vi "Add Topic.vi"(8 "error in (no error)":errorcluster, 9 "Topic Enqueuer":refnum<class "Message Enqueuer.lvclass">, 10 "Topic Object":refnum<class "Topic.lvclass">, 11 "TopicLookupTable":refnum<data-value>) -> (0 "error out":errorcluster, 2 "Topic Replaced?":bool, 3 "TopicLookupTable":refnum<data-value>)   [LabVIEW 2015, in "Mediator.lvlib" / "TopicLookupTable.lvclass"]
doc: "<License>\nCopyright © 2017 Composed Systems, LLC | All rights reserved\nwww.composed.io\n\nAuthor: Ethan Stern <ethan.stern@composed.io>\n\nThis software is provided \"AS IS\" WITHOUT WARRANTIES, either express or implied, AND IS FOR EDUCATIONAL PURPOSES ONLY.\n</License>"
uses:
  TopicLookupTable.lvclass
  Topic/Topic.lvclass
  <vilib>/ActorFramework/Message Enqueuer/Message Enqueuer.lvclass
  Topic/Topic.lvclass/Topic.ctl
  TopicLookupTable.lvclass/TopicLookupTable.ctl
  <vilib>/ErrorRing/Error Ring.xnode
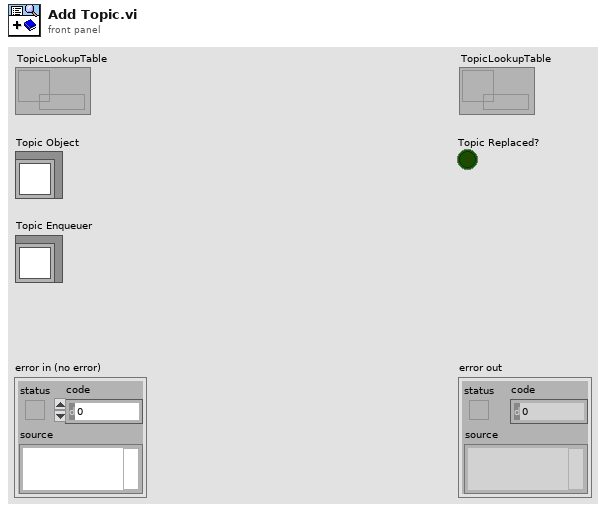
[diagram p1: front panel]
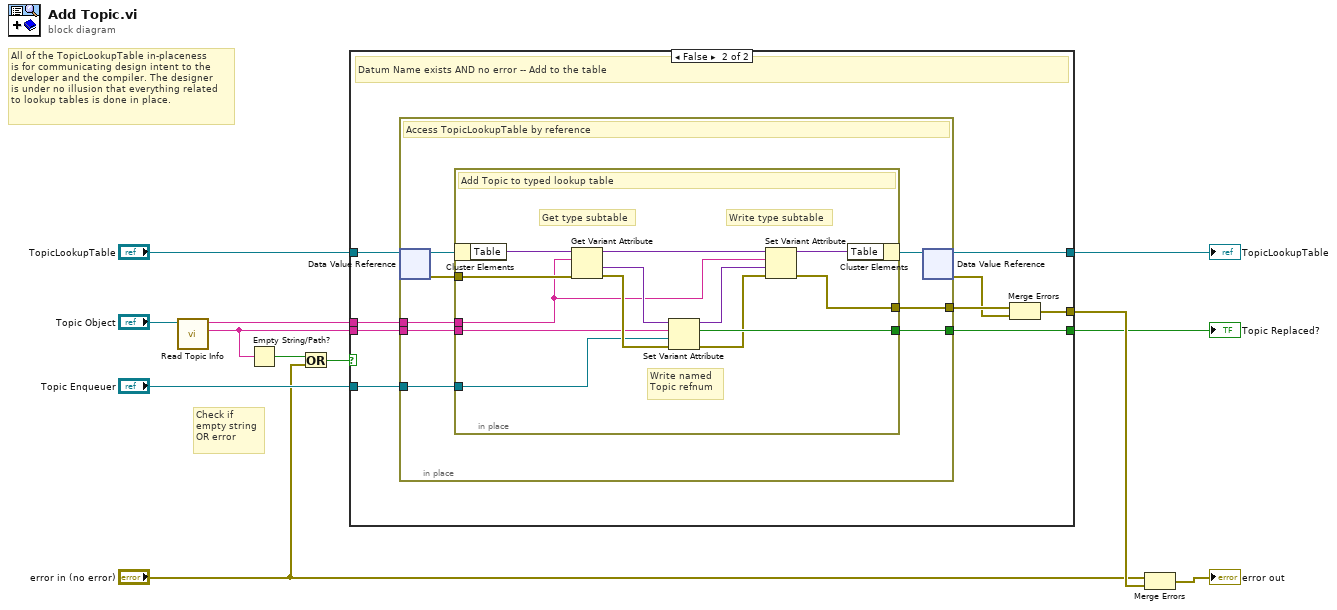
[diagram p0: block diagram]
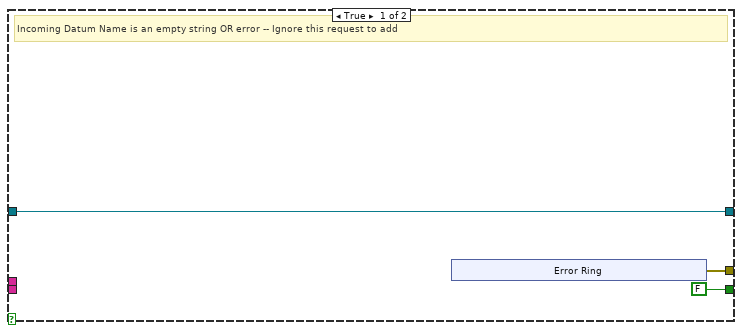
[diagram p2: hidden frame]
diagram:
  # "Check if\nempty string\nOR error"
  # "All of the TopicLookupTable in-placeness\nis for communicating design intent to the\ndeveloper and the compiler. The designer\nis under no illusion that everything related\nto lookup tables is done in place."
  n1 = call "Read Topic Info.vi"("Topic in"="Topic Object") -> ("Name"=w2:string, "Type"=w6:string)  [unwired: 7 in, 2 out]
  n2 = Empty String/Path?(string/path=w2) -> (empty?=w3:bool)
  n3 = Or(x=w3, y="error in (no error)") -> (x .or. y?=w1:bool)
  n4 = case shown="False" w1 {
    tunnel: "TopicLookupTable" -> [w13 w21]
    tunnel: [w14 w20] -> w10
    tunnel: [FALSE ("replaced") w24] -> w9
    tunnel: "Topic Enqueuer" -> [_ w23]
    tunnel: w6 -> [_ w22]
    tunnel: [w13 w18] -> w5
    tunnel: w2 -> [_ w17]
    frame True {
      # "Incoming Datum Name is an empty string OR error -- Ignore this request to add"
      n5 = xnode "Error Ring"() -> ("error out"=w14:errorcluster)
    }
    frame False {
      # "Datum Name exists AND no error -- Add to the table"
      n6 = in-place {
        in-place-border: [w33] -> w25
        in-place-border: [w32] -> w24
        in-place-border: w23 -> [w31]
        in-place-border: w22 -> [w30]
        in-place-border: w17 -> [w29]
        # "Access TopicLookupTable by reference"
        n7 = in-place-dvr #1(w21) -> (w28:refnum<class "TopicLookupTable.lvclass">, w26:errorcluster)
        n8 = in-place {
          in-place-border: [w44] -> w33
          in-place-border: [w39] -> w32
          in-place-border: w31 -> [w37]
          in-place-border: w30 -> [w34]
          in-place-border: w29 -> [w36]
          in-place-border: w26 -> [w35]
          # "Write named\nTopic refnum"
          # "Write type subtable"
          # "Get type subtable"
          # "Add Topic to typed lookup table"
          n9 = in-place-cluster #2(w28) -> ("Table"=w43:variant)
          n10 = Get Variant Attribute(Variant=w43, name=w34, error in=w35) -> (duplicate Variant=w42:variant, value=w40:variant, error out=w46:errorcluster)  [unwired: 1 in, 1 out]
          n11 = Set Variant Attribute(Variant=w40, name=w36, value=w37, error in=w46) -> (Variant out=w41:variant, replaced=w39:bool, error out=w38:errorcluster)
          n12 = Set Variant Attribute(Variant=w42, name=w34, value=w41, error in=w38) -> (Variant out=w45:variant, error out=w44:errorcluster)  [unwired: 1 out]
          n13 = in-place-cluster #2("Table"=w45) -> (w27:refnum<class "TopicLookupTable.lvclass">)
        }
        n14 = in-place-dvr #1(w27) -> (w18:refnum<data-value>, w19:errorcluster)
      }
      n15 = Merge Errors(w25, w19) -> (w20:errorcluster)
    }
  }
  "Topic Replaced?" <- w9
  "TopicLookupTable" <- w5
  n16 = Merge Errors("error in (no error)", w10) -> (→"error out":errorcluster)
